vi "remote.Get Generic Property (Core).vi"(0 "SLSC Remote in":refnum<class "SLSC Interface.lvclass">, 1 "property type":T1, 5 "resources":string, 7 "property":refnum<k21>, 11 "error in (no error)":errorcluster) -> (4 "SLSC Remote out":refnum<class "SLSC Interface.lvclass">, 10 "property value":variant, 15 "error out":errorcluster)   [LabVIEW 2016, in "SLSC Interfaces.lvlib" / "SLSC Interface.lvclass"]
uses:
  SLSC Interface Class/SLSC Interface.lvclass
  <vilib>/NI/NI JSONRPC Server Framework/Classes/Server/JSONRPC Server.lvclass
  <vilib>/httpClient/LabVIEWHTTPClient.lvlib
  <vilib>/httpClient/POSTBuffer.vi
  <vilib>/NI/JSON Support for LabVIEW/JSON Data Classes/JSON Helper/JSON Helper.lvclass
  <vilib>/NI/JSON Support for LabVIEW/JSON Data Classes/JSON Object/JSON Object.lvclass
  <vilib>/NI/JSON Support for LabVIEW/JSON Data Classes/JSON Object/New JSON Object (Empty).vi
  <vilib>/NI/JSON Support for LabVIEW/JSON Data Classes/JSON Object/Insert Key Value Pair (Single String).vi
  <vilib>/NI/NI JSONRPC Server Framework/Classes/Server/Format Client Request (Auto-Increment).vi
  <vilib>/NI/JSON Support for LabVIEW/JSON Data Classes/JSON Object/Get Value (String).vi
  <vilib>/NI/NI JSONRPC Server Framework/Classes/Server/Parse Response (Object).vi
  C:/Program Files (x86)/National Instruments/LabVIEW 2016/vi.lib/NI/JSON Support for LabVIEW/JSON Data Classes/JSON Structured Type/JSON Structure.lvclass
  C:/Program Files (x86)/National Instruments/LabVIEW 2016/vi.lib/NI/JSON Support for LabVIEW/JSON Data Classes/JSON Datatype/JSON Null.lvclass
  <vilib>/NI/JSON Support for LabVIEW/JSON Data Classes/JSON String/JSON String.lvclass
  C:/Program Files (x86)/National Instruments/LabVIEW 2016/vi.lib/NI/JSON Support for LabVIEW/JSON Data Classes/JSON Basic Type/JSON Literal.lvclass
  SLSC Interface Class/Property Type.ctl
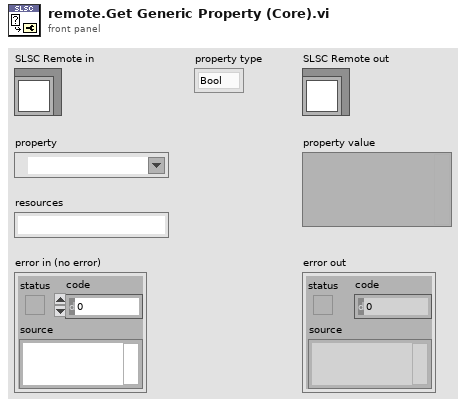
[diagram p1: front panel]
types:
  T1 = typedef "SLSC Interfaces.lvlib/SLSC Interface.lvclass/property type.ctl" = enum16{"Bool", "DBL", "I32", "I64", "String", "U32", "U64", "1D Bool", "1D DBL", "1D I32", "1D I64", "1D String", "1D U32", "1D U64"}
  T2 = typedef "LabVIEWHTTPClient.lvlib/ClientHandle.ctl" = refnum<k1>
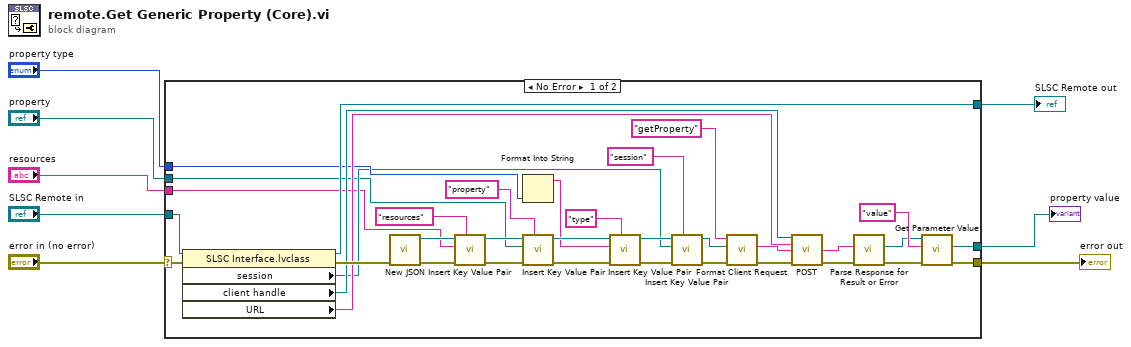
[diagram p0: block diagram]
diagram:
  n1 = case shown="No Error" "error in (no error)" {
    selector: "error in (no error)" -> [w41 w44]
    tunnel: "resources" -> [w10 _]
    tunnel: "SLSC Remote in" -> [w43 w45]
    tunnel: [w42 w45] -> w3
    tunnel: "property" -> [w11 _]
    tunnel: "property type" -> [w26 _]
    tunnel: [w23 w44] -> w2
    tunnel: [w24 _] -> w1
    frame No Error {
      n2 = property class="SLSC Interface.lvclass"(reference=w43, error in=w41) -> (reference out=w42:refnum<class "SLSC Interface.lvclass">, error out=w40:errorcluster, "session"=w12:refnum<k21>, "client handle"=w31:T2, "URL"=w30:string)
      n3 = call-poly <vilib>:"New JSON.vi"("error in (no error)"=w40) -> ("error out"=w39:errorcluster, "JSON Object out"=w21:refnum<class "JSON Object.lvclass">)  [unwired: 9 in]
      n4 = call-poly <vilib>:"Insert Key Value Pair.vi"("key"="resources" ("Name"), "error in (no error)"=w39, "value"=w10, "JSON Object in"=w21) -> ("error out"=w38:errorcluster, "JSON Object out"=w20:refnum<class "JSON Object.lvclass">)  [unwired: 5 in, 1 out]
      n5 = Format Into String(w26) -> (resulting string=w13:string)  [unwired: 3 in, 1 out]
      n6 = call-poly <vilib>:"Insert Key Value Pair.vi"("key"="property" ("Name"), "error in (no error)"=w38, "value"=w11, "JSON Object in"=w20) -> ("error out"=w35:errorcluster, "JSON Object out"=w19:refnum<class "JSON Object.lvclass">)  [unwired: 5 in, 1 out]
      n7 = call-poly <vilib>:"Insert Key Value Pair.vi"("key"="type" ("String"), "error in (no error)"=w35, "value"=w13, "JSON Object in"=w19) -> ("error out"=w34:errorcluster, "JSON Object out"=w18:refnum<class "JSON Object.lvclass">)  [unwired: 5 in, 1 out]
      n8 = call-poly <vilib>:"Insert Key Value Pair.vi"("key"="session" ("Name"), "error in (no error)"=w34, "value"=w12, "JSON Object in"=w18) -> ("error out"=w32:errorcluster, "JSON Object out"=w33:refnum<class "JSON Object.lvclass">)  [unwired: 5 in, 1 out]
      n9 = call-poly <vilib>:"Format Client Request.vi"("error in (no error)"=w32, "JSON in"=w33, "method"="getProperty") -> ("error out"=w29:errorcluster, "Request String"=w36:string)  [unwired: 7 in]
      n10 = call-poly <vilib>:"POST.vi"("client handle"=w31, "url"=w30, "buffer"=w36, "error in (no error)"=w29) -> ("body"=w28:string, "error out"=w27:errorcluster)  [unwired: 8 in, 2 out]
      n11 = call-poly <vilib>:"Parse Response for Result or Error.vi"("error in"=w27, "Response String In"=w28) -> ("error out"=w22:errorcluster, "JSON Array"=w9:refnum<class "JSON Object.lvclass">)  [unwired: 7 in, 1 out]
      n12 = call-poly <vilib>:"Get Parameter Value.vi"("error in (no error)"=w22, "key"="value" ("Parameter Name"), "JSON Object in"=w9) -> ("error out"=w23:errorcluster, "value"=w24:refnum<class "JSON String.lvclass">)  [unwired: 7 in]
    }
    frame Error {
    }
  }
  "error out" <- w2
  "SLSC Remote out" <- w3
  "property value" <- w1
